vi "Add multi-line text to image.vi"(0 "Text to add":string="Insert title text line 1 here\nInsert title text line 2 here\netc.", 1 "Image load path":path, 5 "Text colour":u32(colorbox), 7 "Text position":u16(ring) items=["Top", "Bottom"], 9 "Font, Size & Style":T1={"Desired Font (Application)"=enum."User-specified Font", "[User-specified Font]"={"Font Name"="Arial", "Size"=18, "Strikeout?"=FALSE, "Italic?"=FALSE, "Underline?"=FALSE, "Outline?"=FALSE, "Shadow?"=FALSE, "Bold?"=FALSE, "Rotation Angle"=0.0}, "Horizontal Alignment"=1, "Vertical Alignment"=0} {"Vertical Alignment" items=["Bottom", "Top", "Baseline"]; "Horizontal Alignment" items=["Left", "Center", "Right"]; "[User-specified Font]"."Rotation Angle" format="%.2f"}, 11 "Background colour":u32(colorbox)=16777215, 12 "Image save path":path) -> (15 "Error out":errorcluster)   [LabVIEW 2015]
doc: "Use this VI to add title or caption text to an existing image and then save it to a specified path. The text can be multi-line (simply by having a 'return' (linefeed) character in the string), with options to change the font, size, colour, background colour and font styles."
uses:
  <vilib>/vision/NI_Vision_Development_Module.lvlib
panel:
  out "Image":T2(plugin-control)
  # "PN 25/08/2015"
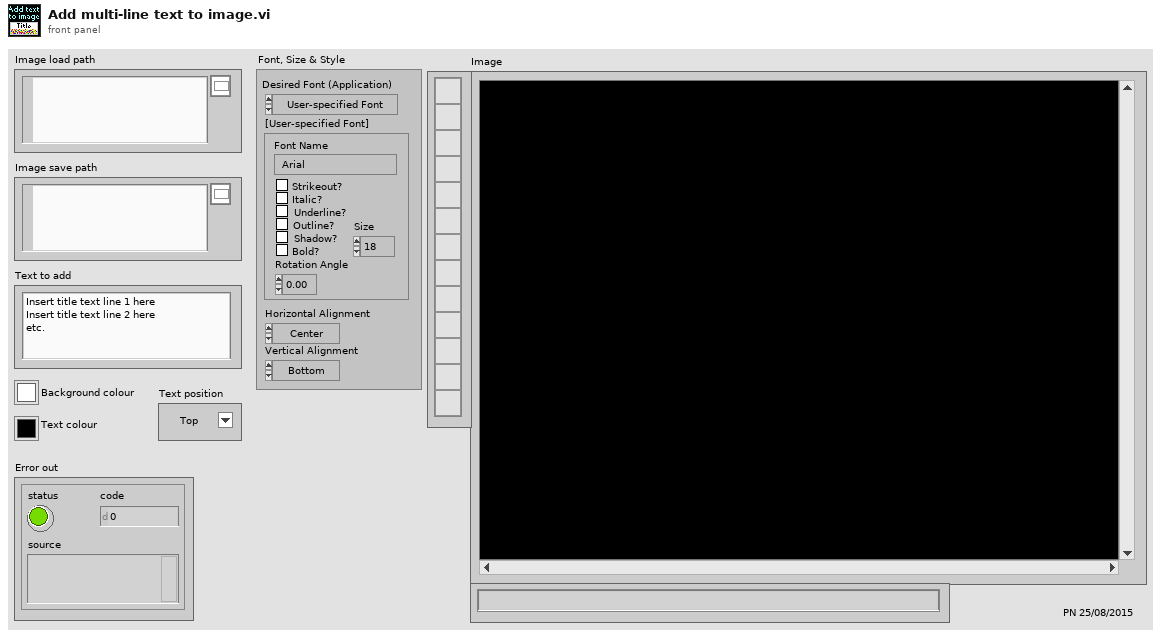
[diagram p1: front panel]
types:
  T1 = cluster{"Desired Font (Application)":enum16{"User-specified Font", "Application Font", "System Font", "Dialog Font"}, "[User-specified Font]":cluster{"Font Name":string, "Size":i16, "Strikeout?":bool, "Italic?":bool, "Underline?":bool, "Outline?":bool, "Shadow?":bool, "Bold?":bool, "Rotation Angle":dbl}, "Horizontal Alignment":i16, "Vertical Alignment":i16}
  T2 = typedef "IMAQ Image.ctl" = refnum<image>
  T3 = cluster{"Left":i32, "Top":i32, "Right":i32, "Bottom":i32}
  T4 = typedef "Image Type" = u32
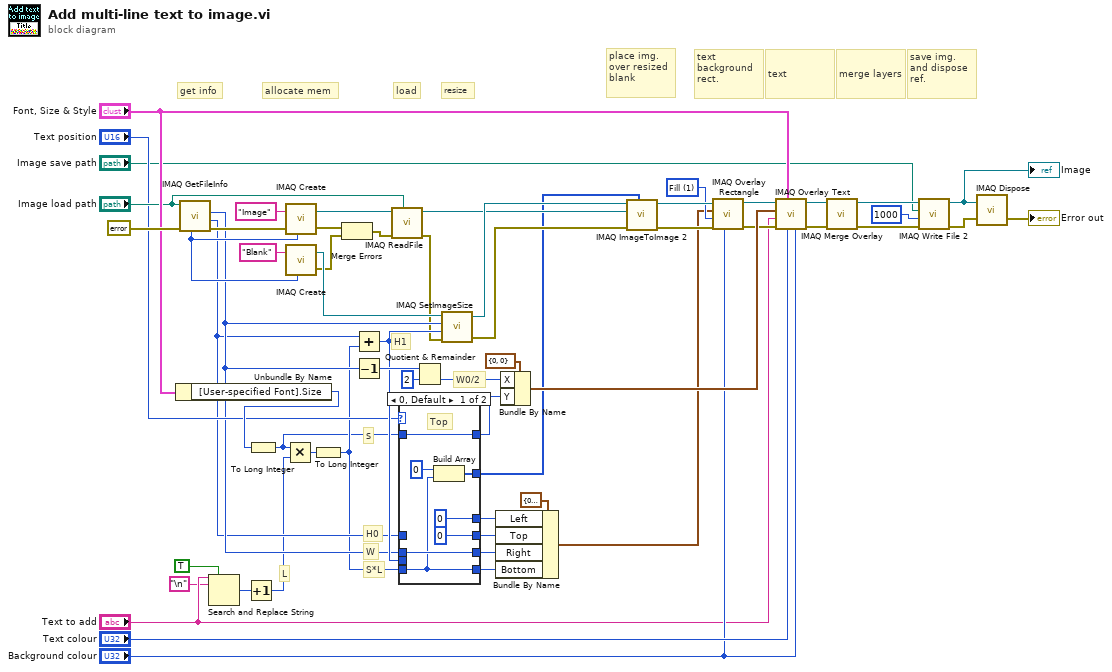
[diagram p0: block diagram]
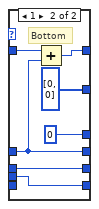
[diagram p2: hidden frame]
diagram:
  w33 = u32 1 items=["Frame", "Fill", "Highlight"] ("Drawing Mode (Frame)")
  # "place img. over resized blank"
  # "resize"
  # "get info"
  # "load"
  # "allocate mem"
  # "W0/2"
  # "H1"
  # "L"
  # "S*L"
  # "S"
  # "W"
  # "H0"
  # "save img. and dispose ref."
  # "merge layers"
  # "text"
  # "text background rect."
  n1 = Unbundle By Name("Font, Size & Style") -> ("[User-specified Font].Size"=w44:i16)
  n2 = call "IMAQ GetFileInfo"("error in (no error)"=errorcluster {"status"=FALSE, "code"=0, "source"=""} ("error in"), "File Path"="Image load path") -> ("error out"=w56:errorcluster, "Y Resolution"=w20:i32, "X Resolution"=w23:i32, "Image Type"=w42:T4)  [unwired: 3 in, 3 out]
  n3 = Search and Replace String(replace all?=TRUE ("replace all? (F)"), input string="Text to add", search string="\n") -> (number of replacements=w10:i32)  [unwired: 5 in, 3 out]
  n4 = Increment(x=w10) -> (x+1=w8:i32)
  n5 = To Long Integer(number=w44) -> (32bit integer=w13:i32)
  n6 = Multiply(x=w13, y=w8) -> (x*y=w47:i32)
  n7 = call "IMAQ Create"("Image Name"="Image", "Image Type"=w42, "error in (no error)"=w56) -> ("New Image"=w41:T2, "error out"=w36:errorcluster)  [unwired: 2 in]
  n8 = call "IMAQ Create"("Image Name"="Blank", "Image Type"=w42) -> ("New Image"=w40:T2, "error out"=w37:errorcluster)  [unwired: 3 in]
  n9 = To Long Integer(number=w47) -> (32bit integer=w14:i32)
  n10 = Merge Errors(w36, w37) -> (w35:errorcluster)
  n11 = Add(x=w20, y=w14) -> (x+y=w29:i32)
  n12 = Decrement(x=w23) -> (x-1=w53:i32)
  n13 = call "IMAQ ReadFile"("File Path"="Image load path", "error in (no error)"=w35, "Image"=w41) -> ("error out"=w19:errorcluster, "Image Out"=w38:T2)  [unwired: 4 in, 3 out]
  n14 = case shown="0, Default" "Text position" {
    tunnel: [w65 w66] -> w30
    tunnel: w13 -> [w65 w67]
    tunnel: w29 -> [_ w70]
    tunnel: [0 ("y") 0 ("y")] -> w25
    tunnel: [0 ("y") w68] -> w24
    tunnel: w23 -> [w62 w71]
    tunnel: [w62 w71] -> w22
    tunnel: w14 -> [w59 _]
    tunnel: [w59 w70] -> w21
    tunnel: w20 -> [_ w68]
    tunnel: [w61 i32[] [0, 0] ("Offset Left/Top")] -> w15
    frame 0, Default {
      # "Top"
      n15 = Build Array(0 ("y"), w59) -> (w61:i32[])
    }
    frame 1 {
      # "Bottom"
      n16 = Add(x=w67, y=w68) -> (x+y=w66:i32)
    }
  }
  n17 = Quotient & Remainder(x=w53, y=2) -> (floor(x/y)=w48:i32)  [unwired: 1 out]
  n18 = call "IMAQ SetImageSize"("error in (no error)"=w19, "Y Resolution"=w29, "X Resolution"=w23, "Image"=w40) -> ("error out"=w18:errorcluster, "Image Out"=w39:T2)  [unwired: 1 in]
  n19 = Bundle By Name(cluster=T3 {"Left"=0, "Top"=0, "Right"=0, "Bottom"=0} ("Rectangle"), "Left"=w25, "Top"=w24, "Right"=w22, "Bottom"=w21) -> (w26:T3)
  n20 = Bundle By Name(cluster=cluster{"X":i32, "Y":i32} {"X"=0, "Y"=0} ("Origin"), "X"=w48, "Y"=w30) -> (w49:cluster{"X":i32, "Y":i32})
  n21 = call "IMAQ ImageToImage 2"("Offset Left/Top"=w15, "error in (no error)"=w18, "Image Src (Small)"=w38, "Image Src (Large)"=w39) -> ("error out"=w32:errorcluster, "Image Dst Out"=w34:T2)  [unwired: 6 in]
  n22 = call "IMAQ Overlay Rectangle"("Color"="Background colour", "error in (no error)"=w32, "Drawing Mode (Frame)"=w33, "Rectangle"=w26, "Image"=w34) -> ("error out"=w16:errorcluster, "Image Out"=w17:T2)  [unwired: 5 in]
  n23 = call "IMAQ Overlay Text"("BG Color (Transparent)"="Background colour", "Text Color (black)"="Text colour", "Font, Size & Style"="Font, Size & Style", "error in (no error)"=w16, "String"="Text to add", "Origin"=w49, "Image"=w17) -> ("error out"=w55:errorcluster, "Image Out"=w45:T2)  [unwired: 3 in]
  n24 = call "IMAQ Merge Overlay"("error in (no error)"=w55, "Image Src"=w45) -> ("error out"=w6:errorcluster, "Image Dst Out"=w7:T2)  [unwired: 8 in]
  n25 = call-poly "IMAQ Write File 2"("error in (no error)"=w6, "Image Quality"=u32 1000, "File Path"="Image save path", "Image"=w7) -> ("error out"=w5:errorcluster, "Image Out (duplicate)"=w3:T2)  [unwired: 6 in]
  "Image" <- w3
  n26 = call "IMAQ Dispose"("Image"=w3, "error in (no error)"=w5) -> ("error out"=→"Error out":errorcluster)  [unwired: 4 in]
